vi "CalculateExperimentTiming.vi"(10 "Experiment":T1={"File Path"=path "", "Operator"="", "Project"="", "Target Dose (dpa)"=0.0, "Sample"={"Name"="", "Description"="", "Molar Mass (g/mol)"=0.0, "Density (g/cm^3)"=0.0, "Irradiation Area (cm^2)"=0.0, "SRIM Damage Peak (disp * ions/cm)"=0.0}, "Beam Line"={"Type"=enum."Ion Beam Analysis", "Ion"=enum."H", "Charge State"=0, "Total Source Ion Energy (kV)"=nan}, "Runs"=[]} {"Beam Line"."Charge State" min=1}, 11 "Calculation Start Time In":timestamp) -> (1 "Duration (sec)":dbl, 2 "Period (sec)":dbl, 3 "Calculation Start Time Out":timestamp)   [LabVIEW 2012]
uses:
  Experiment.ctl
  Sample.ctl
  BeamLine.ctl
  BeamLineType.ctl
  BeamLineIon.ctl
  ExperimentRun.ctl
  ExperimentRunTiming.ctl
  ExperimentRunDose.ctl
  ExperimentRunFluence.ctl
  ExperimentRunTotalCharge.ctl
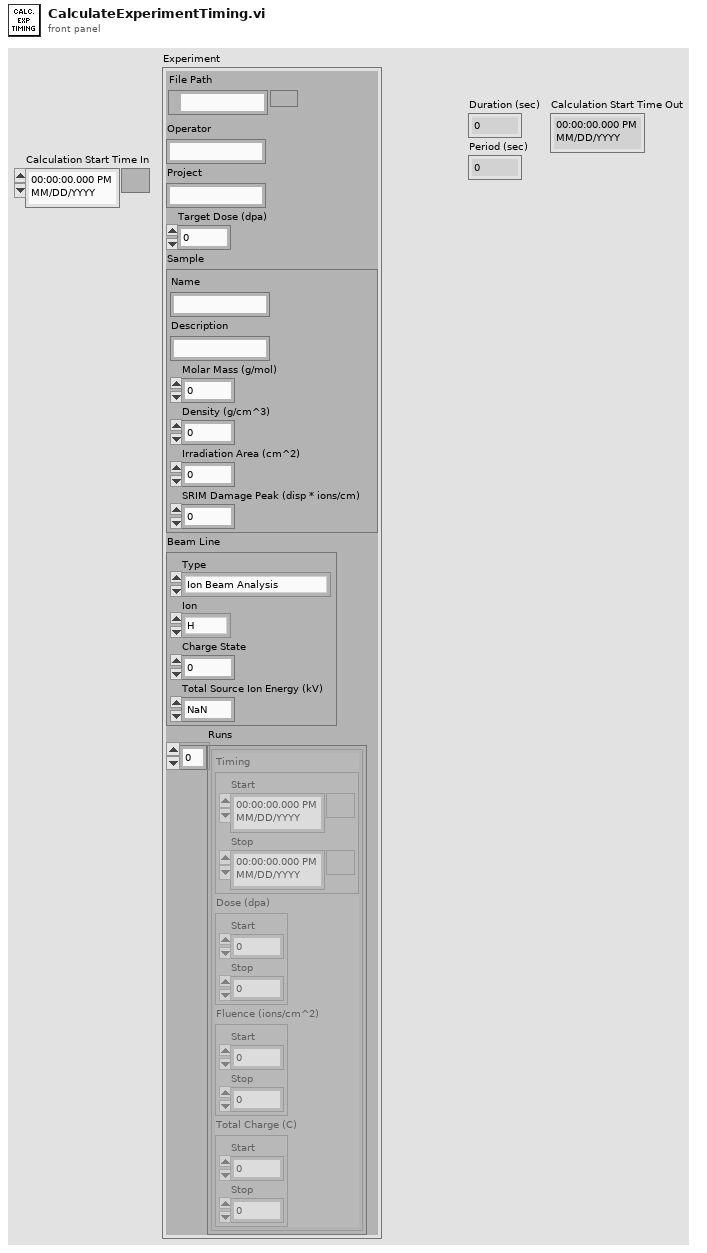
[diagram p1: front panel]
types:
  T1 = typedef "Experiment.ctl" = cluster{"File Path":path, "Operator":string, "Project":string, "Target Dose (dpa)":dbl, "Sample":T2, "Beam Line":T3, "Runs":T6[]}
  T2 = typedef "Sample.ctl" = cluster{"Name":string, "Description":string, "Molar Mass (g/mol)":dbl, "Density (g/cm^3)":dbl, "Irradiation Area (cm^2)":dbl, "SRIM Damage Peak (disp * ions/cm)":dbl}
  T3 = typedef "BeamLine.ctl" = cluster{"Type":T4, "Ion":T5, "Charge State":u8, "Total Source Ion Energy (kV)":dbl}
  T4 = typedef "BeamLineType.ctl" = enum16{"Ion Beam Analysis", "Auxiliary", "Radiation Damage"}
  T5 = typedef "BeamLineIon.ctl" = enum16{"H", "He", "C", "Fe", "Ni", "Pt", "Si", "Ag", "Au"}
  T6 = typedef "ExperimentRun.ctl" = cluster{"Timing":T7, "Dose (dpa)":T8, "Fluence (ions/cm^2)":T9, "Total Charge (C)":T10}
  T7 = typedef "ExperimentRunTiming.ctl" = cluster{"Start":timestamp, "Stop":timestamp}
  T8 = typedef "ExperimentRunDose.ctl" = cluster{"Start":dbl, "Stop":dbl}
  T9 = typedef "ExperimentRunFluence.ctl" = cluster{"Start":dbl, "Stop":dbl}
  T10 = typedef "ExperimentRunTotalCharge.ctl" = cluster{"Start":dbl, "Stop":dbl}
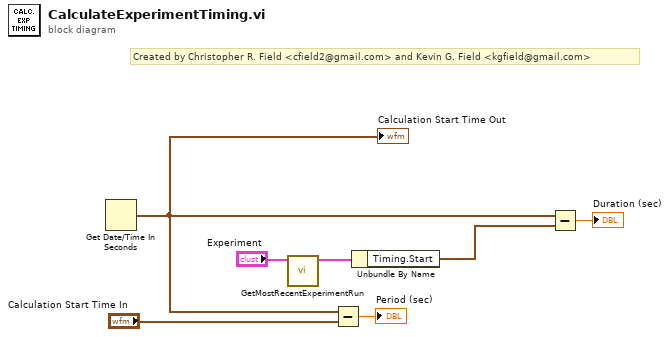
[diagram p0: block diagram]
diagram:
  # "Created by Christopher R. Field <cfield2@gmail.com> and Kevin G. Field <kgfield@gmail.com>"
  n1 = Get Date/Time In Seconds() -> (seconds since 1Jan1904=w6:timestamp)
  "Calculation Start Time Out" <- w6
  n2 = call "GetMostRecentExperimentRun.vi"("Experiment"="Experiment") -> ("Recent Experiment Run"=w2:T6)  [unwired: 10 in]
  n3 = Subtract(x=w6, y="Calculation Start Time In") -> (x-y=→"Period (sec)":dbl)
  n4 = Unbundle By Name(w2) -> ("Timing.Start"=w1:timestamp)
  n5 = Subtract(x=w6, y=w1) -> (x-y=→"Duration (sec)":dbl)
